vi "补齐数据.vi"(9 "总数":i32, 10 "排序后结果输入":string[](array[string]), 11 "數字":string[](array[string])) -> (3 "排序后结果输出":string[](array[string]))   [LabVIEW 2011]
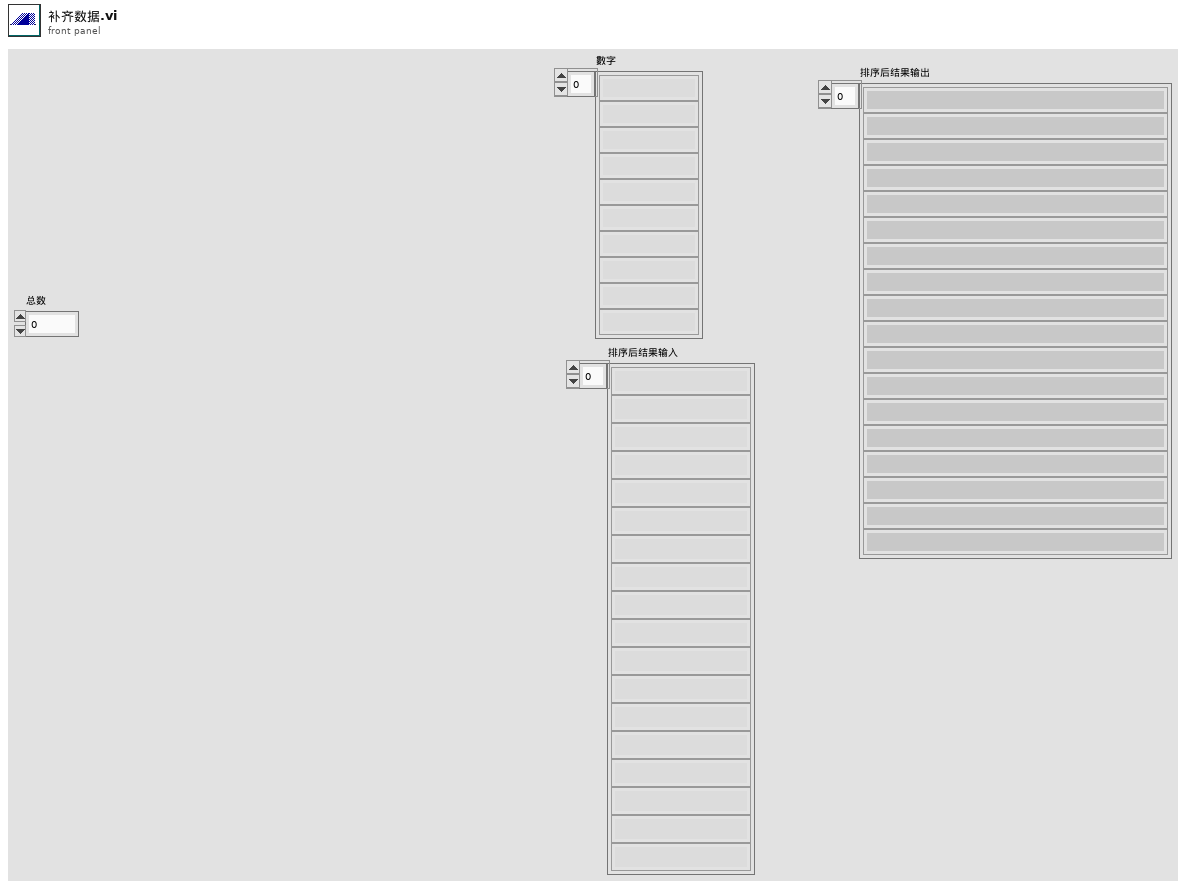
[diagram p1: front panel]
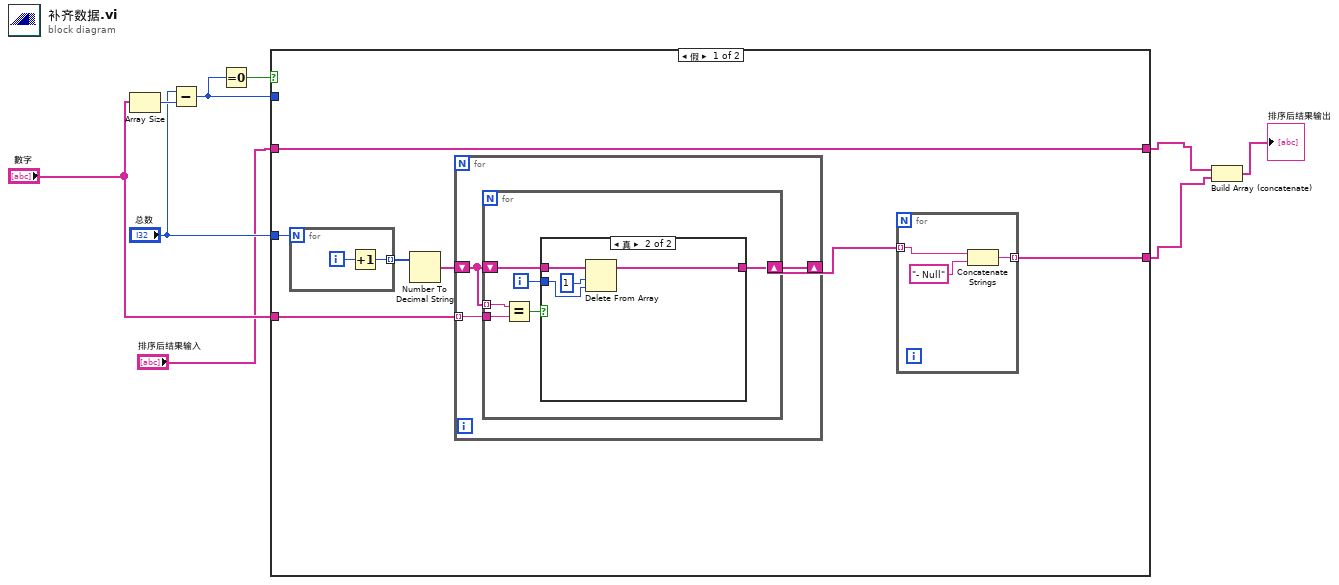
[diagram p0: block diagram]
diagram:
  n1 = Array Size(array="數字") -> (size(s)=w9:i32)
  n2 = Subtract(x="总数", y=w9) -> (x-y=w7:i32)
  n3 = Equal To 0?(x=w7) -> (x = 0?=w8:bool)
  n4 = case shown="假" w8 {
    tunnel: "排序后结果输入" -> [w14 w36]
    tunnel: [w14 w36] -> w3
    tunnel: "數字" -> [w12 _]
    tunnel: w7 -> [_ _]
    tunnel: "总数" -> [w16 _]
    tunnel: [w10 _] -> w2
    frame False {
      n5 = for {
        N: w16 -> [_]
        tunnel: [w34] -> w15 mode=indexing
        i -> [w35]
        n6 = Increment(x=w35) -> (x+1=w34:i32)
      }
      n7 = Number To Decimal String(number=w15) -> (decimal integer string=w13:string[])  [unwired: 1 in]
      n8 = for {
        tunnel: w12 -> [w22] mode=indexing
        shift-right: [w20] -> w11
        shift-left: w13 -> [w21]
        n9 = for {
          tunnel: w21 -> [w28] mode=indexing
          tunnel: w22 -> [w27]
          shift-right: [w23] -> w20
          shift-left: w21 -> [w26]
          i -> [w24]
          n10 = Equal?(x=w28, y=w27) -> (x = y?=w25:bool)
          n11 = case shown="真" w25 {
            tunnel: w26 -> [w29 w33]
            tunnel: w24 -> [_ w32]
            tunnel: [w29 w30] -> w23
            frame False {
            }
            frame True {
              n12 = Delete From Array(array=w33, length=1 ("长度"), index=w32) -> (array with subset deleted=w30:string[])  [unwired: 1 out]
            }
          }
        }
      }
      n13 = for {
        tunnel: w11 -> [w19] mode=indexing
        tunnel: [w17] -> w10 mode=indexing
        n14 = Concatenate Strings(w19, "- Null") -> (w17:string)
      }
    }
    frame True {
    }
  }
  n15 = Build Array (concatenate)(w3, w2) -> (→"排序后结果输出":string[])
